vi "Insert Into Array (String).vi"(8 "error in (no error)":errorcluster, 9 "index":i32, 10 "String":string, 11 "JSON Value in":refnum<class "JSON Value.lvclass">) -> (0 "error out":errorcluster, 3 "JSON Value out":refnum<class "JSON Value.lvclass">)   [LabVIEW 2016, in "JSON Value.lvclass"]
doc: "Inserts an element or subarray into a JSON array at the point you specify in index."
uses:
  JSON Value.lvclass
  Insert Into Array (Value).vi
  New JSON Value/New JSON (String).vi
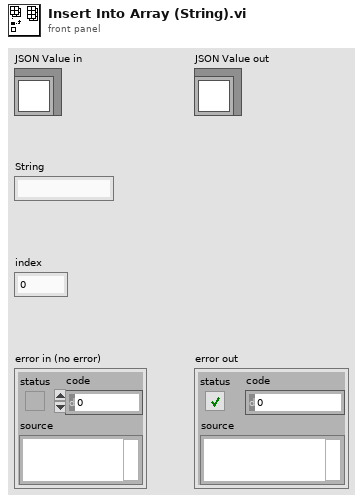
[diagram p1: front panel]
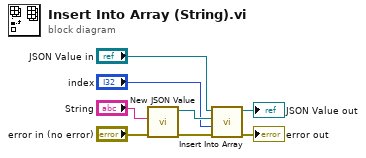
[diagram p0: block diagram]
diagram:
  n1 = call-poly "New JSON Value.vi"("error in (no error)"="error in (no error)", "value"="String") -> ("error out"=w3:errorcluster, "JSON Value out"=w5:refnum<class "JSON Value.lvclass">)  [unwired: 8 in]
  n2 = call-poly "Insert Into Array.vi"("error in (no error)"=w3, "index"="index", 10:"JSON Value in"=w5, 11:"JSON Value in"="JSON Value in") -> ("error out"=→"error out":errorcluster, "JSON Value out"=→"JSON Value out":refnum<class "JSON Value.lvclass">)  [unwired: 6 in]
